vi "MotorTemp_show.vi"(5 "DADES":T1) -> (0 "Temp":dbl, 2 "Cluster":T2, 3 "Button 3":bool, 4 "Button 2":bool, 6 "Button":bool)   [LabVIEW 2018]
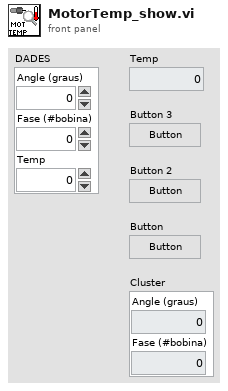
[diagram p1: front panel]
types:
  T1 = cluster{"Angle (graus)":dbl, "Fase (#bobina)":dbl, "Temp":dbl}
  T2 = cluster{"Angle (graus)":dbl, "Fase (#bobina)":dbl}
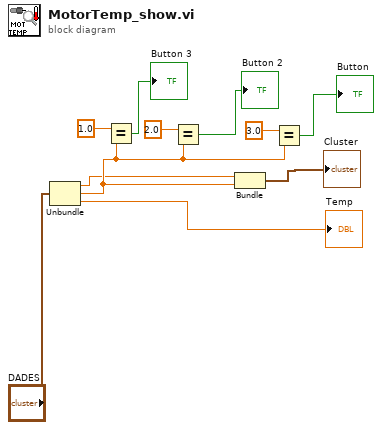
[diagram p0: block diagram]
diagram:
  n1 = Unbundle("DADES") -> ("Angle (graus)"=w8:dbl, "Fase (#bobina)"=w11:dbl, "Temp"=→"Temp":dbl)
  n2 = Equal?(x=1.0, y=w11) -> (x = y?=→"Button 3":bool)
  n3 = Equal?(x=2.0, y=w11) -> (x = y?=→"Button 2":bool)
  n4 = Bundle("Angle (graus)"=w8, "Fase (#bobina)"=w11) -> (→"Cluster":T2)  [unwired: 1 in]
  n5 = Equal?(x=3.0, y=w11) -> (x = y?=→"Button":bool)
